vi "Test App Get Process before and after starting.vi"(8 "error in (no error)":errorcluster, 11 "Rig Test in":refnum<class "Application Test.lvclass">) -> (0 "error out":errorcluster, 3 "Rig Test out":refnum<class "Application Test.lvclass">)   [LabVIEW 2020, in "Application Test.lvclass"]
uses:
  Application Test.lvclass
  C:/Program Files (x86)/National Instruments/LabVIEW 2020/vi.lib/Asteme/LUnit/Test Case.lvclass
  Framework/Process/Process.lvclass
  Framework/Process/Process.lvclass/Process.ctl
  Framework/Application/Application.lvclass/Application.ctl
  <vilib>/Asteme/LUnit/Test Case.lvclass/Test Case.ctl
  <vilib>/Asteme/LUnit/LUnit Assertion Result.lvclass/LUnit Assertion Result.ctl
  Framework/Process/Protected/SubVIs/Set Context.vi
  Framework/Application/Private/Add Process to Map.vi
  Framework/Process/Protected/Messaging/Enqueue Message.vi
  Framework/Process/Public/Get Lifecycle State.vi
  Framework/Process/Protected/Messaging/Request Message.vi
  <vilib>/Asteme/LUnit/Palette/Fail.vi
  <vilib>/Asteme/LUnit/Palette/Pass.vi
  <vilib>/Asteme/LUnit/Set Assertion Type.vi
  Framework/Process/Private/SubVIs/Wait for finish.vi
  Framework/Process/Private/SubVIs/Set Lifecycle State.vi
  <vilib>/Utility/error.llb/Clear Errors.vi
  Framework/Process/Private/SubVIs/Enqueue Request Message.vi
  <vilib>/Asteme/LUnit/Add test result.vi
  <vilib>/Asteme/LUnit/LUnit Write Passed.vi
  <vilib>/Asteme/LUnit/LUnit Get Test Case.vi
  <vilib>/Asteme/LUnit/LUnit Write Message.vi
  <vilib>/Asteme/LUnit/LUnit Write Description.vi
  <vilib>/Asteme/LUnit/LUnit Write Assertion Type.vi
  <vilib>/Asteme/LUnit/Read Test Case Name.vi
  Framework/Application/Application.lvclass
  C:/Users/anton/Documents/GitHub/Triarc-Framework/source/Framework/Process/Process.lvclass
  <vilib>/Utility/error.llb/Error Cluster From Error Code.vi
  Framework/Process/Private/SubVIs/Wait for Response Message.vi
  <vilib>/Asteme/LUnit/Assertion Result/LUnit Get Test Name.vi
  <vilib>/Asteme/LUnit/LUnit Assertion Result.lvclass
  <vilib>/Asteme/LUnit/Test Case.lvclass
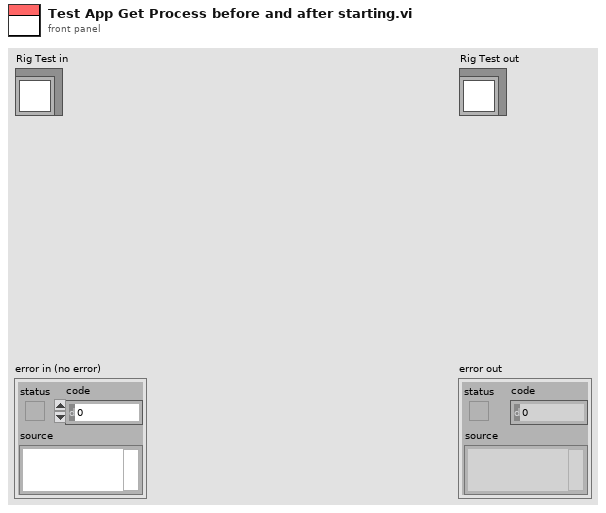
[diagram p1: front panel]
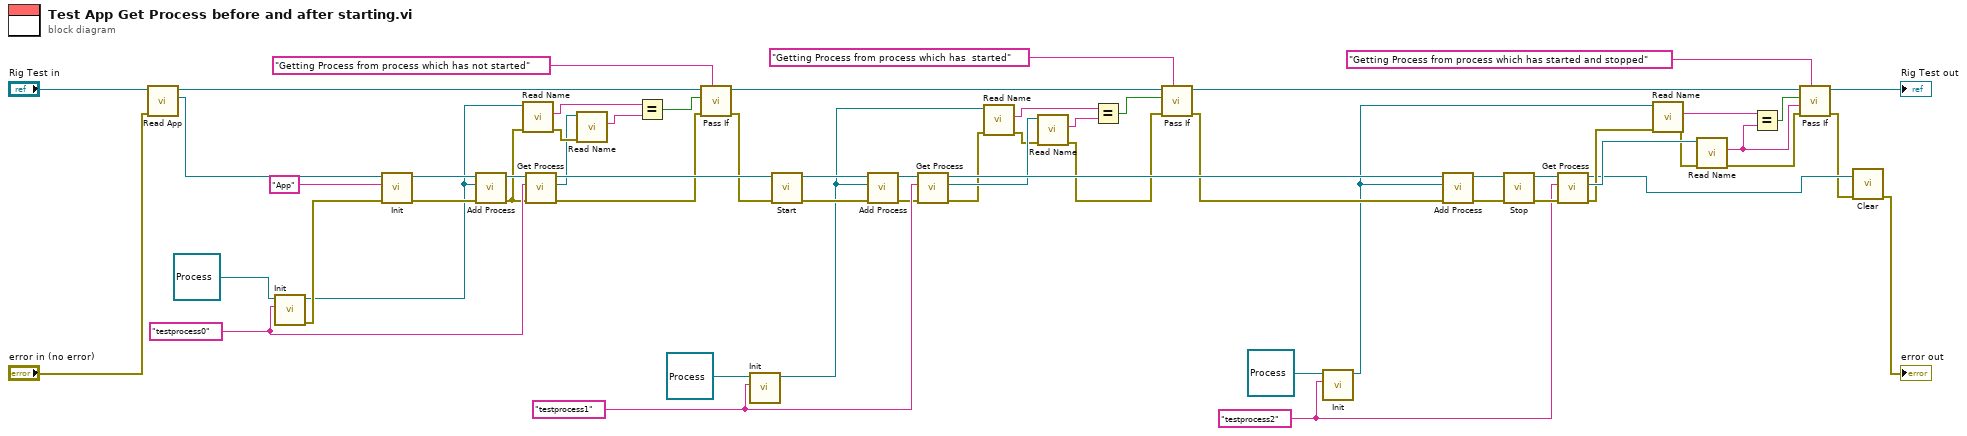
[diagram p0: block diagram]
diagram:
  w32 = "testprocess0" ("Name")
  w44 = "testprocess2" ("Name")
  w52 = "testprocess1" ("Name")
  n1 = call "Read App.vi"("error in (no error)"="error in (no error)", "Application Test In"="Rig Test in") -> ("App out"=w59:refnum<class "Application.lvclass">, "Application Test Out"=w31:refnum<class "Application Test.lvclass">)  [unwired: 7 in, 1 out]
  n2 = call-dynamic "Init.vi"("Name"=w32, "Process In"=refnum<class "Process.lvclass"> refnum ("Process.lvclass")) -> ("error out"=w26:errorcluster, "Process Out"=w5:refnum<class "Process.lvclass">)  [unwired: 8 in]
  n3 = call-dynamic "Init.vi"("error in (no error)"=w26, "Name"="App", "Process In"=w59) -> ("error out"=w34:errorcluster, "Process Out"=w36:refnum<class "Application.lvclass">)  [unwired: 7 in]
  n4 = call "Add Process.vi"("error in (no error)"=w34, "Process"=w5, "Rig In"=w36) -> ("error out"=w1:errorcluster, "Rig Out"=w37:refnum<class "Application.lvclass">)  [unwired: 7 in]
  n5 = call-dynamic "Read Name.vi"("error in (no error)"=w1, "Process In"=w5) -> ("error out"=w7:errorcluster, "Qualified Name"=w4:string)  [unwired: 6 in, 2 out]
  n6 = call "Get Process.vi"("error in (no error)"=w1, "Process Name"=w32, "Rig In"=w37) -> ("error out"=w27:errorcluster, "App Process"=w6:refnum<class "Process.lvclass">, "Rig Out"=w35:refnum<class "Application.lvclass">)  [unwired: 6 in]
  n7 = call-dynamic "Read Name.vi"("error in (no error)"=w7, "Process In"=w6) -> ("Qualified Name"=w3:string)  [unwired: 6 in, 3 out]
  n8 = Equal?(x=w4, y=w3) -> (x = y?=w2:bool)
  n9 = call <vilib>:"Pass If.vi"("Description"="Getting Process from process which has not started", "error in (no error)"=w27, "Pass?"=w2, "Test Case In"=w31) -> ("error out"=w28:errorcluster, "Test Case Out"=w30:refnum<class "Application Test.lvclass">)  [unwired: 6 in]
  n10 = call-dynamic "Init.vi"("Name"=w52, "Process In"=refnum<class "Process.lvclass"> refnum ("Process.lvclass")) -> ("Process Out"=w25:refnum<class "Process.lvclass">)  [unwired: 8 in, 1 out]
  n11 = call "Start.vi"("error in (no error)"=w28, "Process In"=w35) -> ("error out"=w38:errorcluster, "Process Out"=w39:refnum<class "Application.lvclass">)  [unwired: 8 in]
  n12 = call "Add Process.vi"("error in (no error)"=w38, "Process"=w25, "Rig In"=w39) -> ("error out"=w50:errorcluster, "Rig Out"=w54:refnum<class "Application.lvclass">)  [unwired: 7 in]
  n13 = call "Get Process.vi"("error in (no error)"=w50, "Process Name"=w52, "Rig In"=w54) -> ("error out"=w9:errorcluster, "App Process"=w51:refnum<class "Process.lvclass">, "Rig Out"=w56:refnum<class "Application.lvclass">)  [unwired: 6 in]
  n14 = call-dynamic "Read Name.vi"("error in (no error)"=w9, "Process In"=w25) -> ("error out"=w10:errorcluster, "Qualified Name"=w11:string)  [unwired: 6 in, 2 out]
  n15 = call-dynamic "Read Name.vi"("error in (no error)"=w10, "Process In"=w51) -> ("error out"=w8:errorcluster, "Qualified Name"=w12:string)  [unwired: 6 in, 2 out]
  n16 = Equal?(x=w11, y=w12) -> (x = y?=w41:bool)
  n17 = call <vilib>:"Pass If.vi"("Description"="Getting Process from process which has  started", "error in (no error)"=w8, "Pass?"=w41, "Test Case In"=w30) -> ("error out"=w42:errorcluster, "Test Case Out"=w43:refnum<class "Application Test.lvclass">)  [unwired: 6 in]
  n18 = call-dynamic "Init.vi"("Name"=w44, "Process In"=refnum<class "Process.lvclass"> refnum ("Process.lvclass")) -> ("Process Out"=w23:refnum<class "Process.lvclass">)  [unwired: 8 in, 1 out]
  n19 = call "Add Process.vi"("error in (no error)"=w42, "Process"=w23, "Rig In"=w56) -> ("error out"=w47:errorcluster, "Rig Out"=w48:refnum<class "Application.lvclass">)  [unwired: 7 in]
  n20 = call "Stop.vi"("error in (no error)"=w47, "Process In"=w48) -> ("error out"=w45:errorcluster, "Process Out"=w46:refnum<class "Application.lvclass">)  [unwired: 7 in, 1 out]
  n21 = call "Get Process.vi"("error in (no error)"=w45, "Process Name"=w44, "Rig In"=w46) -> ("error out"=w17:errorcluster, "App Process"=w21:refnum<class "Process.lvclass">, "Rig Out"=w15:refnum<class "Application.lvclass">)  [unwired: 6 in]
  n22 = call-dynamic "Read Name.vi"("error in (no error)"=w17, "Process In"=w23) -> ("error out"=w18:errorcluster, "Qualified Name"=w22:string)  [unwired: 6 in, 2 out]
  n23 = call-dynamic "Read Name.vi"("error in (no error)"=w18, "Process In"=w21) -> ("error out"=w16:errorcluster, "Qualified Name"=w19:string)  [unwired: 6 in, 2 out]
  n24 = Equal?(x=w22, y=w19) -> (x = y?=w20:bool)
  n25 = call <vilib>:"Pass If.vi"("Description"="Getting Process from process which has started and stopped", "error in (no error)"=w16, "Message"=w19, "Pass?"=w20, "Test Case In"=w43) -> ("error out"=w14:errorcluster, "Test Case Out"=→"Rig Test out":refnum<class "Application Test.lvclass">)  [unwired: 5 in]
  n26 = call-dynamic "Clear.vi"("error in (no error)"=w14, "Application In"=w15) -> ("error out"=→"error out":errorcluster)  [unwired: 8 in, 1 out]
